vi "PC_reader.vi"() -> ()   [LabVIEW 2019]
panel:
  in  "stop":bool
  out "Sensor value":dbl
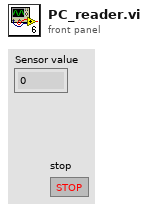
[diagram p1: front panel]
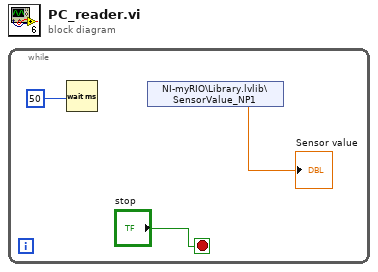
[diagram p0: block diagram]
diagram:
  n1 = while {
    stop <- "stop" stop-if-true
    n2 = Wait (ms)(milliseconds to wait=50) -> ()  [unwired: 1 out]
    n3 = shared-variable "NI-myRIO\\Library.lvlib\\SensorValue_NP1"() -> (→"Sensor value":dbl)  [unwired: 1 in, 1 out]
  }
